vi "Calc Pixel Starting Conditions.vi"(9 "Reciprocals":T6, 11 "Sorted Vertices (V1 is top)":T1={"Top Vertex"={"Position"={"x"=0.0, "y"=0.0, "z"=0.0}, "UV"={"u"=0.0, "v"=0.0}, "Colour"=12517256}, "Mid Vertex"={"Position"={"x"=0.0, "y"=0.0, "z"=0.0}, "UV"={"u"=0.0, "v"=0.0}, "Colour"=12517256}, "Bottom Vertex"={"Position"={"x"=0.0, "y"=0.0, "z"=0.0}, "UV"={"u"=0.0, "v"=0.0}, "Colour"=12517256}, "Alpha"=0.0, "Alpha Blending Enabled"=FALSE} {"Bottom Vertex"."UV"."v" min=0 max=1 step=0.1; "Bottom Vertex"."UV"."u" min=0 max=1 step=0.1; "Mid Vertex"."UV"."v" min=0 max=1 step=0.1; "Mid Vertex"."UV"."u" min=0 max=1 step=0.1; "Top Vertex"."UV"."v" min=0 max=1 step=0.1; "Top Vertex"."UV"."u" min=0 max=1 step=0.1}) -> (3 "Start Row Columns":T5, 5 "Start Row":i32)   [LabVIEW 2022 SP3, in "Raster.lvlib"]
uses:
  Raster.lvlib
  Reciprocals.ctl
  Current Row.ctl
  3D/Triangle (Sorted).ctl
  3D/Vertex.ctl
  3D/Vector 3D.ctl
  UV.ctl
  3D/3D.lvlib
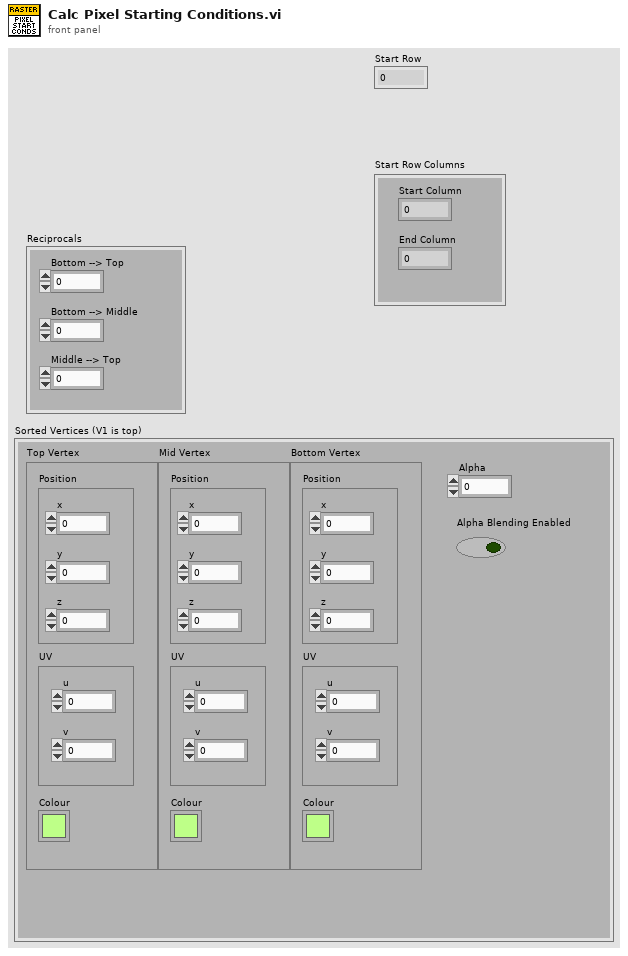
[diagram p1: front panel]
types:
  T1 = typedef "3D.lvlib/Triangle (Sorted).ctl" = cluster{"Top Vertex":T2, "Mid Vertex":T2, "Bottom Vertex":T2, "Alpha":dbl, "Alpha Blending Enabled":bool}
  T2 = typedef "3D.lvlib/Vertex.ctl" = cluster{"Position":T3, "UV":T4, "Colour":u32}
  T3 = typedef "3D.lvlib/Vector 3D.ctl" = cluster{"x":sgl, "y":sgl, "z":sgl}
  T4 = typedef "Raster.lvlib/UV.ctl" = cluster{"u":sgl, "v":sgl}
  T5 = typedef "Raster.lvlib/Current Row.ctl" = cluster{"Start Column":sgl, "End Column":sgl}
  T6 = typedef "Raster.lvlib/Reciprocals.ctl" = cluster{"Bottom --> Top":sgl, "Bottom --> Middle":sgl, "Middle --> Top":sgl}
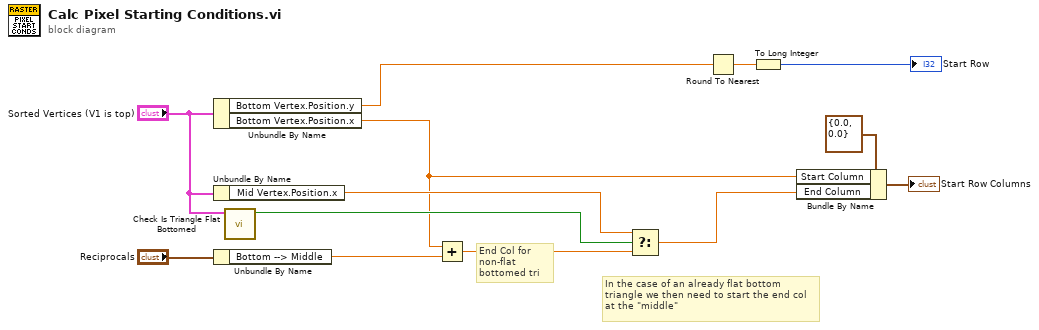
[diagram p0: block diagram]
diagram:
  # "End Col for non-flat bottomed tri"
  # "In the case of an already flat bottom triangle we then need to start the end col at the \"middle\""
  n1 = Unbundle By Name("Sorted Vertices (V1 is top)") -> ("Bottom Vertex.Position.y"=w2:sgl, "Bottom Vertex.Position.x"=w4:sgl)
  n2 = Unbundle By Name("Sorted Vertices (V1 is top)") -> ("Mid Vertex.Position.x"=w6:sgl)
  n3 = Unbundle By Name("Reciprocals") -> ("Bottom --> Middle"=w13:sgl)
  n4 = call "Check Is Triangle Flat Bottomed.vi"("Sorted Triangle"="Sorted Vertices (V1 is top)") -> ("Flat Bottom Triangle"=w7:bool)  [unwired: 10 in]
  n5 = Add(x=w4, y=w13) -> (x+y=w11:sgl)
  n6 = Select(t=w6, s=w7, f=w11) -> (s? t:f=w8:sgl)
  n7 = Round To Nearest(number=w2) -> (nearest integer value=w3:sgl)
  n8 = To Long Integer(number=w3) -> (32bit integer=→"Start Row":i32)
  n9 = Bundle By Name(cluster=T5 {"Start Column"=0.0, "End Column"=0.0} ("Current Row"), "Start Column"=w4, "End Column"=w8) -> (→"Start Row Columns":T5)
